vi "Server.vi"() -> ()   [LabVIEW 2014]
doc: "Demonstrates how to set up a basic TCP connection, send data to the specified port once a connection has been established, and terminate the connection once the data has been sent. This VI is designed to stop if the TCP connection is terminated. The data sent in this example is an array of random numbers."
uses:
  <vilib>/sound2/lvsound2.llb/Sound Data Format.ctl
  <vilib>/sound2/lvsound2.llb/Sound Input Read (DBL).vi
  <vilib>/Waveform/WDTOps.llb/WDT Index Channel DBL.vi
panel:
  out "data string":string
  out "waveform":waveform(dbl)
  in  "Stop":bool
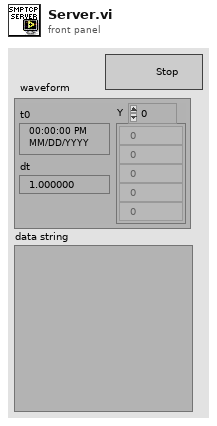
[diagram p1: front panel]
types:
  T1 = typedef "Sound Data Format.ctl" = cluster{"sample rate (S/s)":dbl, "number of channels":i32, "bits per sample":i32}
  T2 = typedef "Sound Input Task ID.ctl" = u32
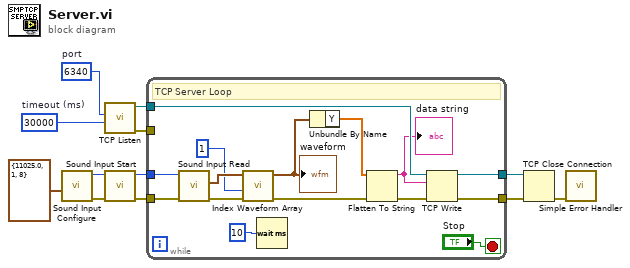
[diagram p0: block diagram]
diagram:
  w6 = u16 6340  # port
  w7 = 30000  # timeout (ms)
  n1 = call <vilib>:"Sound Input Configure.vi"("sound format"=T1 {"sample rate (S/s)"=11025.0, "number of channels"=1, "bits per sample"=8}) -> ("error out"=w3:errorcluster, "task ID"=w4:T2)  [unwired: 9 in]
  n2 = call <vilib>:"TCP Listen.vi"("timeout ms (wait forever: -1)"=w7, "port"=w6) -> ("error out"=w8:errorcluster, "connection ID"=w9:refnum<k5>)  [unwired: 5 in, 3 out]
  n3 = call <vilib>:"Sound Input Start.vi"("error in (no error)"=w3, "task ID"=w4) -> ("error out"=w1:errorcluster, "task ID out"=w2:T2)  [unwired: 8 in]
  n4 = while {
    tunnel: [w26] -> w11
    tunnel: [w24] -> w12
    tunnel: w9 -> [w23]
    tunnel: w8 -> [_]
    tunnel: w2 -> [w21]
    tunnel: w1 -> [w20]
    stop <- "Stop" stop-if-true
    # "TCP Server Loop"
    n5 = call-poly <vilib>:"Sound Input Read.vi"("error in (no error)"=w20, "task ID"=w21) -> ("error out"=w19:errorcluster, "data"=w17:waveform(dbl)[])  [unwired: 7 in, 1 out]
    n6 = call-poly <vilib>:"Index Waveform Array.vi"("error in (no error)"=w19, "index"=1, "waveform array"=w17) -> ("error out"=w18:errorcluster, "waveform"=w16:waveform(dbl))  [unwired: 7 in]
    "waveform" <- w16
    n7 = Wait (ms)(milliseconds to wait=u32 10) -> ()  [unwired: 1 out]
    n8 = Unbundle By Name(w16) -> ("Y"=w15:dbl[])
    n9 = Flatten To String(anything=w15, error in (no error)=w18) -> (data string=w13:string, error out=w22:errorcluster)  [unwired: 2 in, 1 out]
    "data string" <- w13
    n10 = TCP Write(connection ID=w23, data in=w13, error in (no error)=w22) -> (connection ID out=w24:refnum<k5>, error out=w26:errorcluster)  [unwired: 2 out]
  }
  n11 = TCP Close Connection(connection ID=w12, error in (no error)=w11) -> (error out=w10:errorcluster)  [unwired: 2 out]
  n12 = call <vilib>:"Simple Error Handler.vi"("error in (no error)"=w10) -> ()  [unwired: 1 in, 8 out]
